vi "Error Cluster From First Error Status Bit.vi"(8 "error in (no error)":errorcluster, 11 "VISA resource name":refnum<visa-resource-name>) -> (0 "error out":errorcluster, 3 "VISA resource name out":refnum<visa-resource-name>)   [LabVIEW 2013, in "SRS SR400.lvlib"]
doc: "Checks all error status bits and creates an error cluster from the first bit that is enabled, if any.\n\nThis VI uses Error Cluster From Error Status Bit.vi to check each status bit. Refer to that VI's documentation for further information."
uses:
  <instrlib>/SRS SR400/SRS SR400.lvlib
  <instrlib>/SRS SR400/Public/Typedefs/Error Codes Matrix.ctl
  <instrlib>/SRS SR400/Public/Typedefs/Error Status Bit.ctl
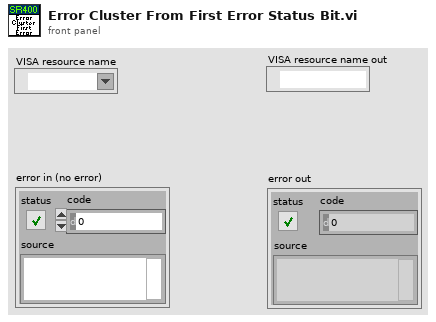
[diagram p1: front panel]
types:
  T1 = typedef "SRS SR400.lvlib/Error Codes Matrix.ctl" = string[][]
  T2 = typedef "SRS SR400.lvlib/Error Status Bit.ctl" = u16
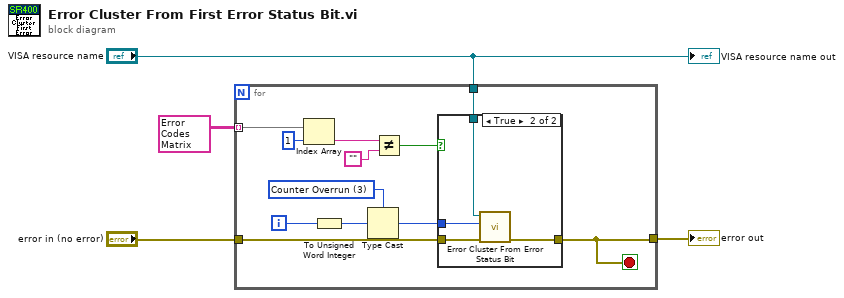
[diagram p0: block diagram]
diagram:
  n1 = for {
    tunnel: T1 [["", ""], ["", ""], ["", ""], ["3", "Counter Overrun. This bit is set whenever counter A or B exceeds or equals 10^9 - 1 counts."], ["4", "Rate Error. This bit is set whenever a gate is missed. This can occur if a gate delay or width exceeds the trigger period minus 1 µs."], ["5", "Recall Error. This bit is set if a recall from a stored setting detects an error in the recalled data. If an error is found, the instrument setup is not altered."], ["", ""], ["7", "Command Error. This bit is set when an illegal command is received."]] ("Error Codes Matrix") -> [w13] mode=indexing
    tunnel: "error in (no error)" -> [w7]
    tunnel: [w5] -> w2
    tunnel: "VISA resource name" -> [w6]
    i -> [w16]
    stop <- w5 stop-if-true
    w14 = T2 3 items=["Counter Overrun"=3, "Rate Error"=4, "Recall Error"=5, "Command Error"=7] ("Error Status Bit (Command Error)")
    n2 = Index Array(array=w13, index=1) -> (element=w8:string)
    n3 = To Unsigned Word Integer(number=w16) -> (unsigned 16bit integer=w15:u16)
    n4 = Type Cast(type=w14, x=w15) -> (*(type *) &x=w9:T2)
    n5 = Not Equal?(x=w8, y="") -> (x != y?=w10:bool)
    n6 = case shown="True" w10 {
      tunnel: w9 -> [_ w21]
      tunnel: w7 -> [w17 w20]
      tunnel: [w17 w19] -> w5
      tunnel: w6 -> [_ w18]
      frame False {
      }
      frame True {
        n7 = call <instrlib>:"Error Cluster From Error Status Bit.vi"("error in (no error)"=w20, "Error Status Bit (Command Error)"=w21, "VISA resource name"=w18) -> ("error out"=w19:errorcluster)  [unwired: 7 in, 1 out]
      }
    }
  }
  "error out" <- w2
  "VISA resource name out" <- "VISA resource name"
